vi "QR Code_Release.vi"(8 "error in":errorcluster, 11 "Buffer Data":T1) -> (0 "error out":errorcluster)   [LabVIEW 2016]
uses:
  Data Def/QR Code_Buffer Data.ctl
  <vilib>/vision/Image Controls.llb/IMAQ Image.ctl
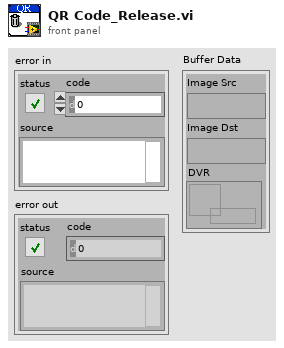
[diagram p1: front panel]
types:
  T1 = typedef "QR Code_Buffer Data.ctl" = cluster{"Image Src":T2, "Image Dst":T2, "DVR":refnum<data-value>}
  T2 = typedef "IMAQ Image.ctl" = refnum<image>
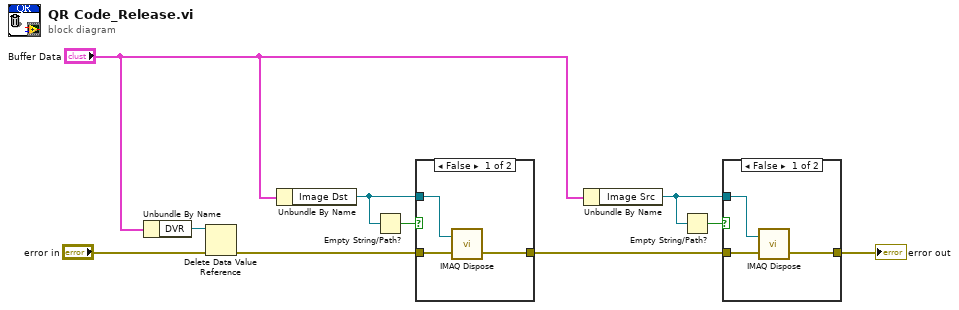
[diagram p0: block diagram]
diagram:
  n1 = Unbundle By Name("Buffer Data") -> ("DVR"=w2:refnum<data-value>)
  n2 = Delete Data Value Reference(data value reference=w2, error in="error in") -> (error out=w1:errorcluster)  [unwired: 1 out]
  n3 = Unbundle By Name("Buffer Data") -> ("Image Dst"=w9:T2)
  n4 = Empty String/Path?(string/path=w9) -> (empty?=w10:bool)
  n5 = case shown="False" w10 {
    tunnel: w9 -> [w13 _]
    tunnel: w1 -> [w12 w14]
    tunnel: [w11 w14] -> w6
    frame False {
      n6 = call "IMAQ Dispose"("Image"=w13, "error in (no error)"=w12) -> ("error out"=w11:errorcluster)  [unwired: 4 in]
    }
    frame True {
    }
  }
  n7 = Unbundle By Name("Buffer Data") -> ("Image Src"=w8:T2)
  n8 = Empty String/Path?(string/path=w8) -> (empty?=w7:bool)
  n9 = case shown="False" w7 {
    tunnel: w8 -> [w17 _]
    tunnel: w6 -> [w16 w18]
    tunnel: [w15 w18] -> w5
    frame False {
      n10 = call "IMAQ Dispose"("Image"=w17, "error in (no error)"=w16) -> ("error out"=w15:errorcluster)  [unwired: 4 in]
    }
    frame True {
    }
  }
  "error out" <- w5
